vi "Read trigger holdoff (500.0 E-9 s).vi"(8 "error in (no error)":errorcluster, 11 "Configure Trigger Msg in":refnum<class "Configure Trigger Msg.lvclass">) -> (0 "error out":errorcluster, 2 "trigger holdoff (500.0 E-9 s)":dbl[unit]=5e-07 format="%^.2e", 3 "Configure Trigger Msg out":refnum<class "Configure Trigger Msg.lvclass">)   [LabVIEW 2015, in "CS++Scope.lvlib" / "Configure Trigger Msg.lvclass"]
uses:
  Configure Trigger Msg.lvclass
  Configure Trigger Msg.lvclass/Configure Trigger Msg.ctl
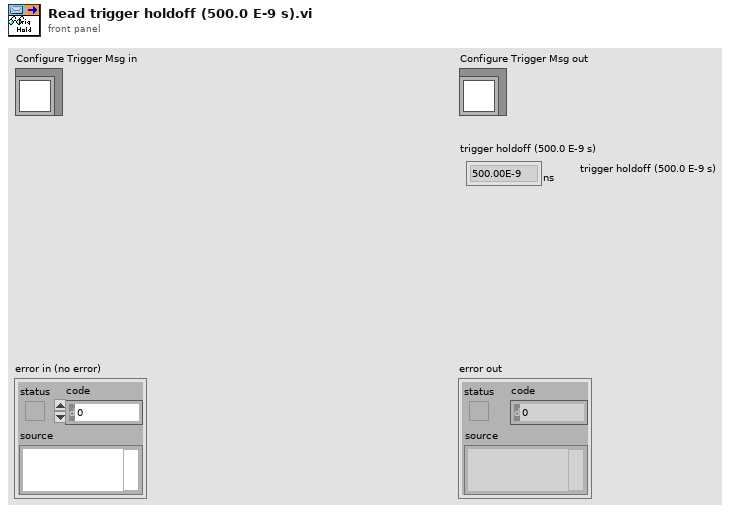
[diagram p1: front panel]
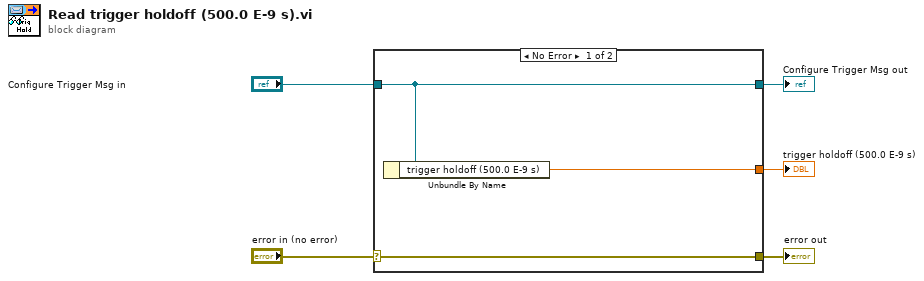
[diagram p0: block diagram]
diagram:
  n1 = case shown="No Error" "error in (no error)" {
    selector: "error in (no error)" -> [w8 w9]
    tunnel: [w8 w9] -> w4
    tunnel: [w7 w10] -> w2
    tunnel: "Configure Trigger Msg in" -> [w7 w10]
    tunnel: [w6 _] -> w1
    frame No Error {
      n2 = Unbundle By Name(w7) -> ("trigger holdoff (500.0 E-9 s)"=w6:dbl[unit])
    }
    frame Error {
    }
  }
  "error out" <- w4
  "Configure Trigger Msg out" <- w2
  "trigger holdoff (500.0 E-9 s)" <- w1
